vi "Extract Channel Data.vi"(10 "module configuration":refnum<class "fixed channel tag bus module configuration.lvclass">, 11 "Engine Configuration":refnum<class "engine configuration.lvclass">) -> (1 "Channel Data":string[][](array[string]), 2 "module configuration out":refnum<class "fixed channel tag bus module configuration.lvclass">, 3 "Engine Configuration Out":refnum<class "engine configuration.lvclass">)   [LabVIEW 2013, in "fixed channel tag bus module editor node.lvclass"]
uses:
  fixed channel tag bus module editor node.lvclass
  <vilib>/NI/Module Execution Interface/Engine Configuration/engine configuration.lvclass
  module/configuration/fixed channel tag bus module configuration.lvclass
  <vilib>/NI/Tag Bus Module Framework/root configuration/TBM configuration.lvclass/TBM configuration.ctl
  <vilib>/NI/Tag Bus/tag/tag descriptor.lvclass/tag descriptor.ctl
  <vilib>/NI/Tag Bus Module Framework/channel/TBM channel.lvclass/TBM channel.ctl
  <vilib>/NI/Tag Bus Module Framework/root configuration/create GUID.vi
  <vilib>/NI/Tag Bus/tag/tag descriptor.lvclass
  <vilib>/NI/Tag Bus Module Framework/root configuration/TBM configuration.lvclass
  <vilib>/NI/Tag Bus Module Framework/channel/TBM channel.lvclass
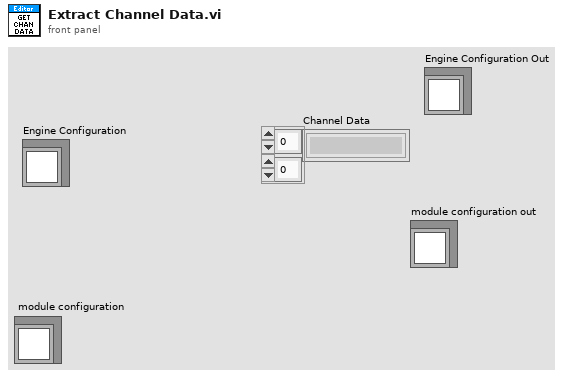
[diagram p1: front panel]
types:
  T1 = typedef "TBM channel.lvclass/channel classification.ctl" = enum16{"input data", "output data", "processing parameter", "processing result"}
  T2 = typedef "tag bus.lvlib/tag descriptor.lvclass/Data Type.ctl" = enum16{"Double", "Single", "I64", "I32", "I16", "I8", "U64", "U32", "U16", "U8", "Boolean", "String", "Array of Double", "Array of Single", "Array of I64", "Array of I32", "Array of I16", "Array of I8", "Array of U64", "Array of U32", "Array of U16", "Array of U8", "Array of Boolean", "Array of String"}
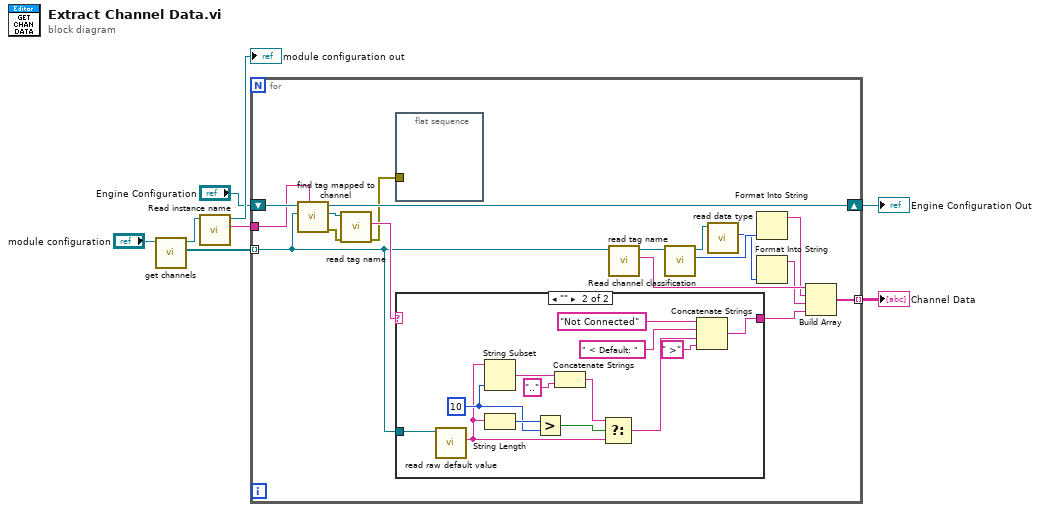
[diagram p0: block diagram]
diagram:
  n1 = call-dynamic "get channels.vi"("user tag bus module configuration In"="module configuration") -> ("channels"=w1:refnum<class "TBM channel.lvclass">[], "user tag bus module configuration Out"=w2:refnum<class "fixed channel tag bus module configuration.lvclass">)  [unwired: 9 in]
  n2 = call <vilib>:"Read instance name.vi"("configuration in"=w2) -> ("instance id"=w6:string, "configuration out"=→"module configuration out":refnum<class "fixed channel tag bus module configuration.lvclass">)  [unwired: 8 in, 1 out]
  n3 = for {
    tunnel: w1 -> [w16] mode=indexing
    tunnel: [w23] -> w8 mode=indexing
    tunnel: w6 -> [w22]
    shift-right: [w20] -> w3
    shift-left: "Engine Configuration" -> [w25]
    n4 = call <vilib>:"find tag mapped to channel.vi"("owner"=w22, "channel"=w16, "engine configuration in"=w25) -> ("error out"=w21:errorcluster, "tag"=w24:refnum<class "tag descriptor.lvclass">, "engine configuration out"=w20:refnum<class "engine configuration.lvclass">)  [unwired: 6 in]
    n5 = call <vilib>:"read tag name.vi"("error in"=w21, "system tag in"=w24) -> ("error out"=w17:errorcluster, "name"=w19:string)  [unwired: 7 in, 1 out]
    n6 = flat-sequence {
      tunnel: w17 -> [_]
      frame #0 {
      }
    }
    n7 = case shown="\"\"" w19 {
      selector: w19 -> [w26 _]
      tunnel: [w26 w27] -> w18
      tunnel: w16 -> [_ w29]
      frame Default {
      }
      frame "" {
        w35 = 10 ("y")
        n8 = call <vilib>:"read raw default value.vi"("system tag in"=w29) -> ("raw default"=w31:string)  [unwired: 8 in, 2 out]
        n9 = String Subset(string=w31, length (rest)=w35) -> (substring=w33:string)  [unwired: 1 in]
        n10 = String Length(string=w31) -> (length=w37:i32)
        n11 = Greater?(x=w37, y=w35) -> (0:w36:bool)
        n12 = Concatenate Strings(w33, ".." ("string")) -> (w34:string)
        n13 = Select(t=w34, s=w36, f=w31) -> (s? t:f=w30:string)
        n14 = Concatenate Strings("Not Connected", " < Default: " ("string"), w30, " >" ("string")) -> (w27:string)
      }
    }
    n15 = call <vilib>:"read tag name.vi"("system tag in"=w16) -> ("name"=w15:string, "system tag out"=w9:refnum<class "TBM channel.lvclass">)  [unwired: 8 in, 1 out]
    n16 = call <vilib>:"Read channel classification.vi"("channel in"=w9) -> ("channel classification"=w14:T1, "channel out"=w11:refnum<class "TBM channel.lvclass">)  [unwired: 8 in, 1 out]
    n17 = call <vilib>:"read data type.vi"("system tag in"=w11) -> ("data type"=w10:T2)  [unwired: 8 in, 2 out]
    n18 = Format Into String(w14) -> (resulting string=w13:string)  [unwired: 3 in, 1 out]
    n19 = Format Into String(w10) -> (resulting string=w12:string)  [unwired: 3 in, 1 out]
    n20 = Build Array(w15, w13, w12, w18) -> (w23:string[])
  }
  "Channel Data" <- w8
  "Engine Configuration Out" <- w3
